vi "CreateWindow.vi"(8 "error in (no error)":errorcluster, 11 "Window in":refnum<class "Window.lvclass">) -> (0 "error out":errorcluster, 2 "Window [SDL_Window *]":i64, 3 "Window out":refnum<class "Window.lvclass">)   [LabVIEW 2024, in "GLF.lvlib" / "Window.lvclass"]
uses:
  Window.lvclass
  Window.lvclass/Window.ctl
  <vilib>/Saukko/LV SDL3/Sources/SDL3/Video/Video.lvlib
  <vilib>/Saukko/LV SDL3/Sources/SDL3/Video/WindowFlags--ring.ctl
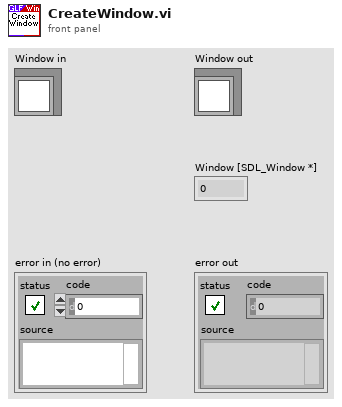
[diagram p1: front panel]
types:
  T1 = typedef "SDL3.lvlib/Video.lvlib/WindowFlags--ring.ctl" = u64
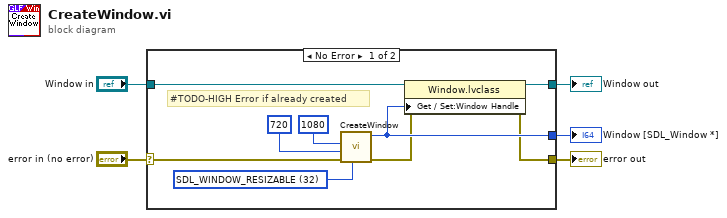
[diagram p0: block diagram]
diagram:
  n1 = case shown="No Error" "error in (no error)" {
    selector: "error in (no error)" -> [w14 w16]
    tunnel: [w6 w16] -> w4
    tunnel: [w9 w15] -> w2
    tunnel: "Window in" -> [w10 w15]
    tunnel: [w8 _] -> w1
    frame No Error {
      w11 = T1 32 items=["0"=0, "SDL_WINDOW_FULLSCREEN"=1, "SDL_WINDOW_OPENGL"=2, "SDL_WINDOW_OCCLUDED"=4, "SDL_WINDOW_HIDDEN"=8, "SDL_WINDOW_BORDERLESS"=16, "SDL_WINDOW_RESIZABLE"=32, "SDL_WINDOW_MINIMIZED"=64, "SDL_WINDOW_MAXIMIZED"=128, "SDL_WINDOW_MOUSE_GRABBED"=256, "SDL_WINDOW_INPUT_FOCUS"=512, "SDL_WINDOW_MOUSE_FOCUS"=1024, "SDL_WINDOW_EXTERNAL"=2048, "SDL_WINDOW_MODAL"=4096, "SDL_WINDOW_HIGH_PIXEL_DENSITY"=8192, "SDL_WINDOW_MOUSE_CAPTURE"=16384, "SDL_WINDOW_MOUSE_RELATIVE_MODE"=32768, "SDL_WINDOW_ALWAYS_ON_TOP"=65536, "SDL_WINDOW_UTILITY"=131072, "SDL_WINDOW_TOOLTIP"=262144, "SDL_WINDOW_POPUP_MENU"=524288, "SDL_WINDOW_KEYBOARD_GRABBED"=1048576, "SDL_WINDOW_VULKAN"=268435456, "SDL_WINDOW_METAL"=536870912, "SDL_WINDOW_TRANSPARENT"=1073741824, "SDL_WINDOW_NOT_FOCUSABLE"=2147483648] ("flags (0)")
      # "#TODO-HIGH Error if already created"
      n2 = call <vilib>:"CreateWindow.vi"("Flags (0)"=w11, "No Error"=w14, "h"=720, "w"=1080) -> ("Error Out"=w7:errorcluster, "Window [SDL_Window *]"=w8:i64)  [unwired: 6 in]
      n3 = property class="Window.lvclass"(reference=w10, error in=w7, "Get / Set:Window Handle"=w8) -> (reference out=w9:refnum<class "Window.lvclass">, error out=w6:errorcluster)
    }
    frame Error {
    }
  }
  "error out" <- w4
  "Window out" <- w2
  "Window [SDL_Window *]" <- w1
